vi "append alias to string.vi"(9 "alias":string[](array[string]), 10 "dev name \"space\" var name":string[](array[string]), 11 "Channel name in in":string) -> (3 "Channel name out":string)   [LabVIEW 2020]
uses:
  MySQL/Preset Query Enum.ctl
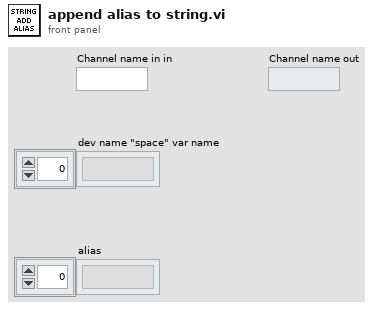
[diagram p1: front panel]
types:
  T1 = typedef "Preset Query Enum.ctl" = enum16{"Get Locations", "Get all IPs and MACs", "Get classes", "Get expt variables to set at scanstart for particular device", "Get expt devices and variables with start values", "Get expt devices and variables (with data to get)", "Get expt devices with data to get", "Get Expt devices and GUIs", "Get all devices basic properties", "Get Virtual Devices Core Info", "Get Expt names", "Get experiment basic properties", "Get experiment alarm variables", "Get MC Ports", "Get device network comm port", "Get devicetype lvclass path", "Get basic device properties", "Get Init Order", "Get all setable variables of a device", "Get device variable aliases", "Get force values of all settable variables", "Get all variables of a devicetype", "Get all variables of a device", "Get plotter details", "Get Saved Scans", "Get Scan Info", "GetGeneralGUIs", "Get expt for plotter", "Get plotter IDs from expt", "Get all devices", "Get all Virtual Devices", "Get all aliases", "Get variable and device info for Virtual Device", "GetItemLocatorIP", "Get IPs for GUIs", "Get DeviceType from Device", "GetLocalPortRange", "GetDevicePresetVariables", "Get Device Configuration", "GetAllPresetNames", "GetAllConfigurationNames", "GetPresetDeviceNames", "GetDeviceAliases", "GetDevicesOfClass"}
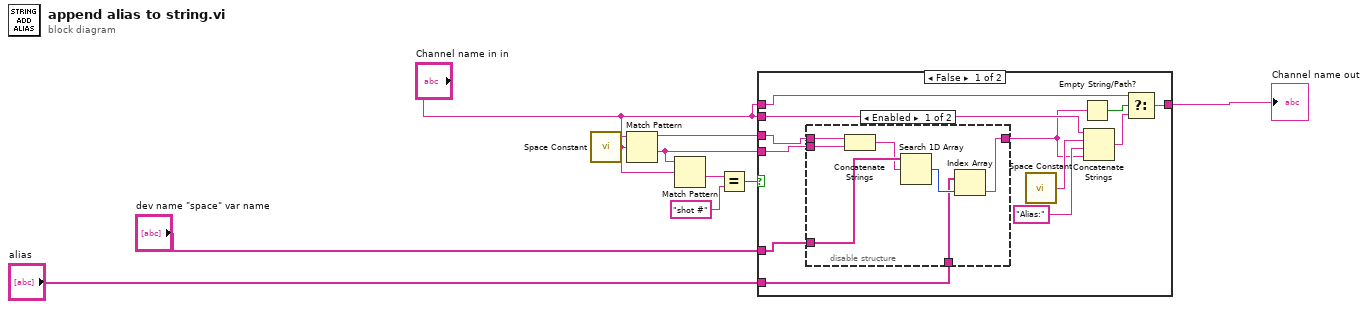
[diagram p0: block diagram]
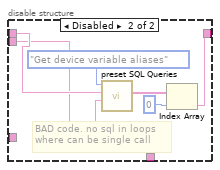
[diagram p2: hidden frame]
diagram:
  n1 = call <vilib>:"Space Constant.vi"() -> ("String"=w4:string)
  n2 = Match Pattern(string="Channel name in in", regular expression=w4) -> (before substring=w9:string, after substring=w8:string)  [unwired: 1 in, 2 out]
  n3 = Match Pattern(string=w8, regular expression=w4) -> (after substring=w5:string)  [unwired: 1 in, 3 out]
  n4 = Equal?(x=w5, y="shot #") -> (x = y?=w7:bool)
  n5 = case shown="False" w7 {
    tunnel: [w20 w36] -> w10
    tunnel: "Channel name in in" -> [w21 w36]
    tunnel: "Channel name in in" -> [w19 _]
    tunnel: w8 -> [w14 _]
    tunnel: w9 -> [w15 _]
    tunnel: "dev name \"space\" var name" -> [w13 _]
    tunnel: "alias" -> [w12 _]
    frame False {
      n6 = disable-structure shown="Enabled" {
        disable-tunnel: w15 -> [w29 w32]
        disable-tunnel: w14 -> [w28 w31]
        disable-tunnel: w13 -> [w27 _]
        disable-tunnel: w12 -> [w24 _]
        disable-tunnel: [w23 w30] -> w11
        frame Enabled {
          n7 = Concatenate Strings(w29, w28) -> (w26:string)
          n8 = Search 1D Array(1D array=w27, element=w26) -> (index of element=w25:i32)  [unwired: 1 in]
          n9 = Index Array(array=w24, index=w25) -> (element=w23:string)
        }
        frame Disabled {
          # "BAD code. no sql in loops\nwhere can be single call"
          n10 = call "preset SQL Queries.vi"("Expt name / MCIP/ Variable/Preset Name"=w31, "Device/Devicetype name\n/Plotter.id/ScanName#"=w32, "Preset Query"=Preset_Query_Enum."Get device variable aliases") -> ("1st column 1st data"=w35:string[])  [unwired: 6 in, 2 out]
          n11 = Index Array(array=w35, index=0) -> (element=w30:string)
        }
      }
      n12 = call <vilib>:"Space Constant.vi"() -> ("String"=w18:string)
      n13 = Empty String/Path?(string/path=w11) -> (empty?=w22:bool)
      n14 = Concatenate Strings(w19, w18, "Alias:" ("string"), w11) -> (w17:string)
      n15 = Select(t=w21, s=w22, f=w17) -> (s? t:f=w20:string)
    }
    frame True {
    }
  }
  "Channel name out" <- w10
